vi "Image Imencode And Imdecode.vi"() -> ()   [LabVIEW 2018]
doc: "Image Imencode And Imdecode: This example is an example of encoding and decoding images, which encodes image data into a specific format byte stream for transmission or storage, and can decode these encoded byte streams into the original image data. Through image encoding and decoding, the transmission, storage, and processing of image data, as well as image interaction and interoperability between different systems, can be achieved."
uses:
  vi.lib/VIRobotics/opencv_yiku/Mat/Mat_8U/Mat_8U.lvclass
  D:/Program Files/company/National Instruments/LabVIEW 2018/vi.lib/addons/VIRobotics/opencv_yiku/Mat/Mat/Mat.lvclass
  vi.lib/VIRobotics/opencv_yiku/opencv_yiku.lvlib
  vi.lib/VIRobotics/opencv_yiku/Mat/Mat/Mat.lvclass
panel:
  out "size(s)":i32
  out "length":i32
  in  "quality":i32=50
  out "picture":picture
  # "Overview: Demonstrates how to encode and save an image to the local system, and then decode and restore it back to the image format by reading the local file.\nRequirements: Windows.\nInstructions: \n1. Run the VI."
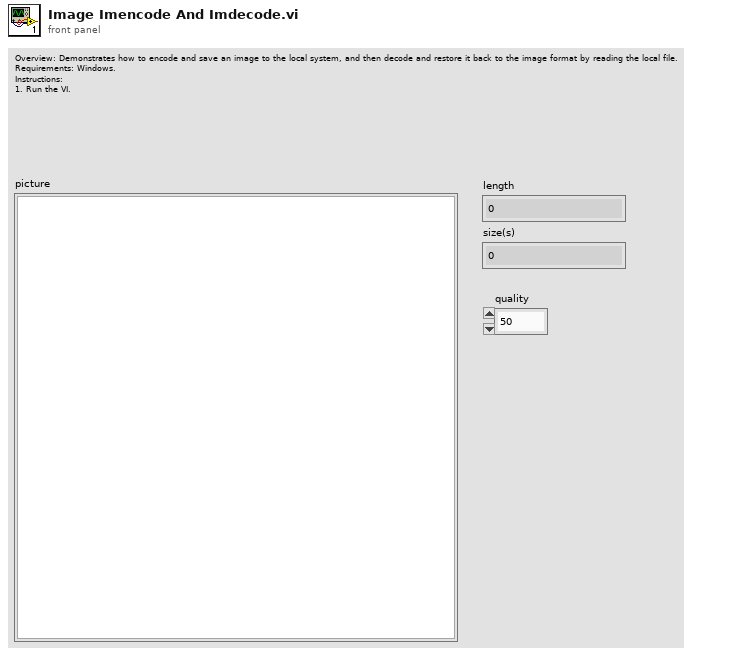
[diagram p1: front panel]
types:
  T1 = enum16{"open", "replace", "create", "open or create", "replace or create", "replace or create with confirmation"}
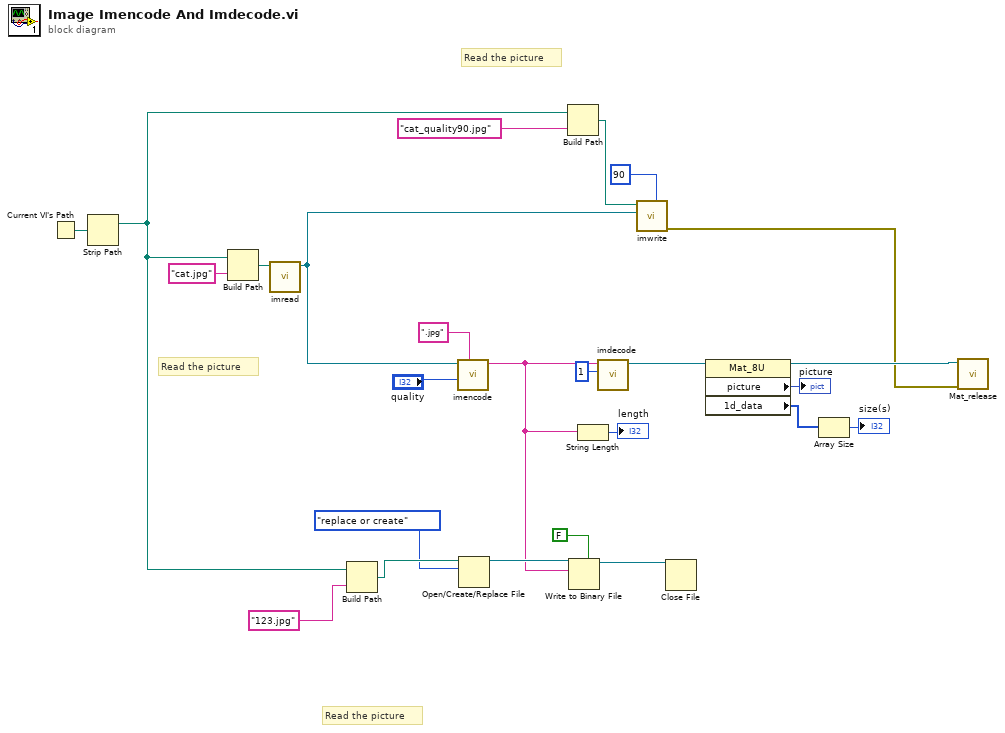
[diagram p0: block diagram]
diagram:
  # "Read the picture"
  # "Read the picture"
  # "Read the picture"
  n1 = Current VI's Path() -> (path=w25:path)
  n2 = Strip Path(path=w25) -> (stripped path=w1:path)  [unwired: 1 out]
  n3 = Build Path(base path=w1, name or relative path="cat.jpg") -> (appended path=w24:path)
  n4 = call "imread.vi"("path"=w24) -> ("Mat out"=w3:refnum<class "Mat_8U.lvclass">)  [unwired: 9 in, 1 out]
  n5 = Build Path(base path=w1, name or relative path="123.jpg") -> (appended path=w21:path)
  n6 = call "imencode.vi"("exte"=".jpg", "quality"="quality", "Mat out"=w3) -> ("bytes"=w11:string)  [unwired: 7 in, 1 out]
  n7 = Open/Create/Replace File(file path (use dialog)=w21, operation (0:open)=T1."replace or create") -> (refnum out=w19:refnum<file>)  [unwired: 4 in, 2 out]
  n8 = Build Path(base path=w1, name or relative path="cat_quality90.jpg") -> (appended path=w6:path)
  n9 = Write to Binary File(file (use dialog)=w19, data=w11, 5:FALSE ("prepend array or string size? (T)")) -> (refnum out=w17:refnum<file>)  [unwired: 3 in, 2 out]
  n10 = String Length(string=w11) -> (length=→"length":i32)
  n11 = call "imdecode.vi"("flag"=1, "String"=w11) -> ("Mat out"=w15:refnum<class "Mat_8U.lvclass">)  [unwired: 8 in, 1 out]
  n12 = call "imwrite.vi"("quality"=90, "Mat out"=w3, "path"=w6) -> ("error out"=w4:errorcluster)  [unwired: 8 in]
  n13 = Close File(refnum=w17) -> ()  [unwired: 1 in, 2 out]
  n14 = property class="Mat_8U"(reference=w15) -> (reference out=w5:refnum<class "Mat_8U.lvclass">, "picture"=→"picture":picture, "1d_data"=w9:u8[])  [unwired: 1 in, 1 out]
  n15 = Array Size(array=w9) -> (size(s)=→"size(s)":i32)
  n16 = call "Mat_release.vi"("error in (no error)"=w4, "Mat in"=w5) -> ()  [unwired: 9 in, 1 out]
